vi "Read configuration.vi"(8 "error in":errorcluster, 11 "Modbus Slave editor node in":refnum<class "Modbus Slave editor node.lvclass">) -> (0 "error out":errorcluster, 2 "configuration":refnum<class "NISE_CEF_serializable configuration.lvclass">, 3 "Modbus Slave editor node out":refnum<class "Modbus Slave editor node.lvclass">)   [LabVIEW 2013, in "Modbus Slave editor node.lvclass"]
doc: "Platypus Framework 1.0.1.65\nNI Systems Engineering - National Instruments"
uses:
  Modbus Slave editor node.lvclass
  <vilib>/NI/Configuration Framework/serializable configuration/NISE_CEF_serializable configuration.lvclass
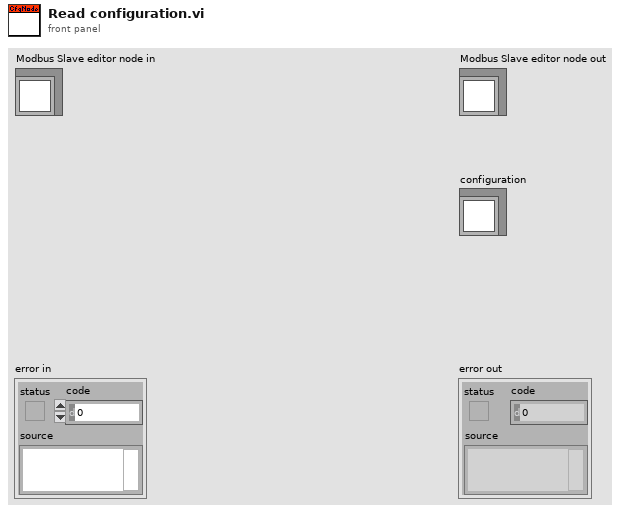
[diagram p1: front panel]
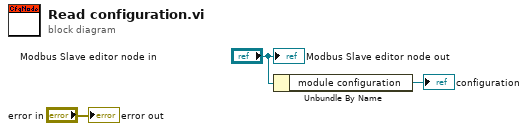
[diagram p0: block diagram]
diagram:
  n1 = Unbundle By Name("Modbus Slave editor node in") -> ("module configuration"=→"configuration":refnum<class "Modbus Slave configuration.lvclass">)
  "error out" <- "error in"
  "Modbus Slave editor node out" <- "Modbus Slave editor node in"
